vi "PH_AxisGUI_BaseClass.PC Stop.vi"(0 "VI in":refnum<vi>, 5 "error in (no error)":errorcluster) -> (14 "VI out":refnum<vi>, 19 "error out":errorcluster)   [LabVIEW 2014, in "PH_AxisGUI_BaseClass.lvlib"]
doc: "This VI acts on an axis."
uses:
  PH_AxisGUI_BaseClass.lvlib
  PH_Stepmotor_BaseClass/PH_Stepmotor_BaseClass.lvlib
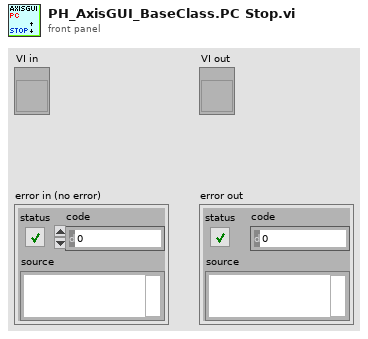
[diagram p1: front panel]
types:
  T1 = typedef "PH_AxisGUI_BaseClass.lvlib/PH_AxisGUI_BaseClass.i attribute.ctl" = cluster{"Axes":T2[]}
  T2 = typedef "PH_AxisGUI_BaseClass.lvlib/PH_AxisGUI_BaseClass.Axis Attributes.ctl" = cluster{"Axis GUI Refs":T3, "Address":T4, "Name":string, "Label \"Back\"":string, "Labell \"Forth\"":string, "Moving?":bool}
  T3 = typedef "PH_AxisGUI_BaseClass.lvlib/PH_AxisGUI_BaseClass.Axis GUI Refs.ctl" = cluster{"Back":refnum<vi>, "Forth":refnum<vi>, "Status":refnum<vi>, "Target":refnum<vi>, "Address":refnum<vi>, "Status Bar":refnum<vi>, "Settings":refnum<vi>, "Activity":refnum<vi>, "Clear Error":refnum<vi>}
  T4 = typedef "PH_Stepmotor_BaseClass.lvlib/PH_Stepmotor_BaseClass.Axis Address.ctl" = cluster{"Instance":string, "Motor Nr":i32}
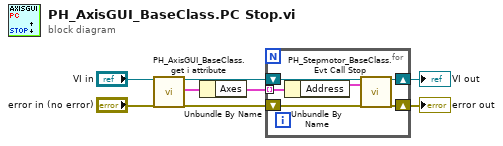
[diagram p0: block diagram]
diagram:
  n1 = call "PH_AxisGUI_BaseClass.get i attribute.vi"("i ref in"="VI in", "error in (no error)"="error in (no error)") -> ("i ref out"=w6:refnum<vi>, "i attribute"=w2:T1, "error out"=w4:errorcluster)  [unwired: 15 in]
  n2 = Unbundle By Name(w2) -> ("Axes"=w1:T2[])
  n3 = for {
    tunnel: w1 -> [w10] mode=indexing
    shift-right: [w13] -> w7
    shift-left: w6 -> [w12]
    shift-right: [w14] -> w8
    shift-left: w4 -> [w11]
    n4 = Unbundle By Name(w10) -> ("Address"=w9:T4)
    n5 = call "PH_Stepmotor_BaseClass.Evt Call Stop.vi"("i ref in"=w12, "Address"=w9, "error in"=w11) -> ("i ref out"=w13:refnum<vi>, "error out"=w14:errorcluster)  [unwired: 15 in]
  }
  "error out" <- w8
  "VI out" <- w7
